vi "R567X_CAN高级功能.vi"(0 "Function":T1(ring), 11 "error in":errorcluster) -> (2 "当前扭矩":dbl, 3 "当前角度":dbl, 4 "完成":bool, 6 "Out_Time":bool, 8 "角度已标定":bool, 10 "扭矩已标定":bool, 15 "error out":errorcluster)   [LabVIEW 2020]
uses:
  Global_Variable/Global.vi
  Libraries/ZLG_CAN/ZLG_CAN.lvlib
  Libraries/S7/S7.lvlib
panel:
  out "Logs":string
  in  "CAN 通道":u32(ring) items=["0", "1"]
  in  "设备类型":u32(ring)=27 items=["PCI5121"=1, "PCI9810"=2, "USBCAN1"=3, "USBCAN2"=4, "PCI9820"=5, "PCI5110"=7, "PC104CAN"=11, "CANETUDP"=12, "PCI9840B"=14, "PC104C2"=15, "PCI9820I"=16, "CANETTCP"=17, "PCIE9221"=24, "PCI5010U"=19, "USBCAN_E_U"=20, "USBCAN_2E_U"=21, "PCI5020U"=22, "PCIE9120I"=27, "PCIE9110I"=28, "PCIE9140I"=29]
  in  "索引":u32(ring) items=["0", "1", "2", "3", "4", "5", "6", "7", "8"]
  in  "波特率":u32(ring)=11 items=["5Kbps", "10Kbps", "20Kbps", "40Kbps", "50Kbps", "80Kbps", "100Kbps", "125Kbps", "200Kbps", "250Kbps", "400Kbps", "500Kbps", "666Kbps", "800Kbps", "1000Kbps"]
  out "B'":i16 format="%x"
  out "B":i16 format="%x"
  out "A":i16 format="%x"
  out "A'":i16 format="%x"
  out "标定成功":bool caption="启动标定成功"
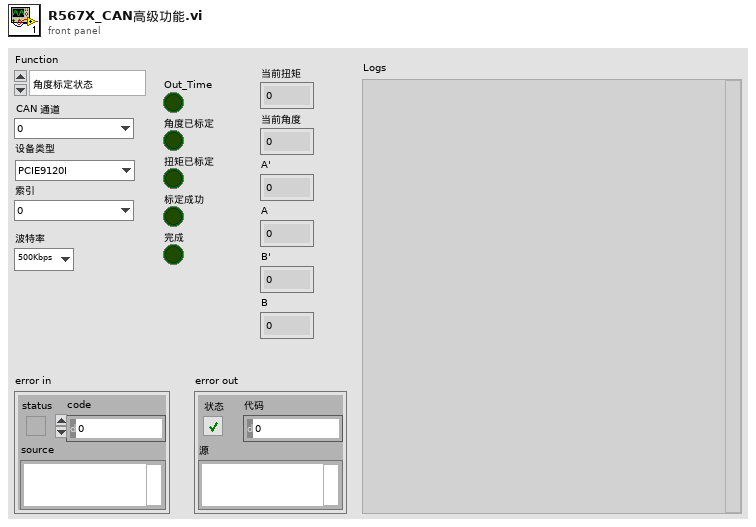
[diagram p1: front panel]
types:
  T1 = enum16{"角度标定状态", "角度标定", "角度标定清除", "扭矩标定状态", "扭矩标定", "扭矩标定清除", "内部软件版本号", "客户软件版本号"}
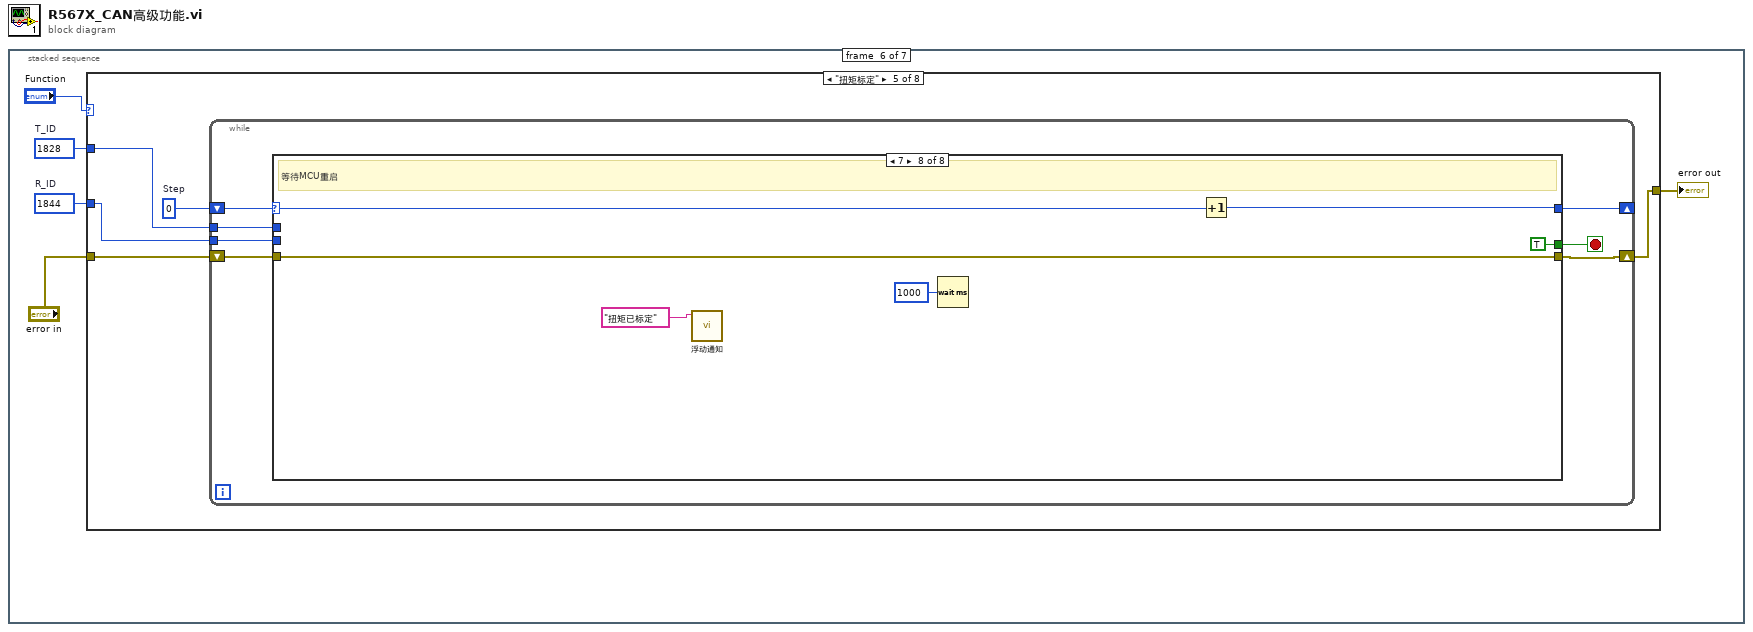
[diagram p0: block diagram]
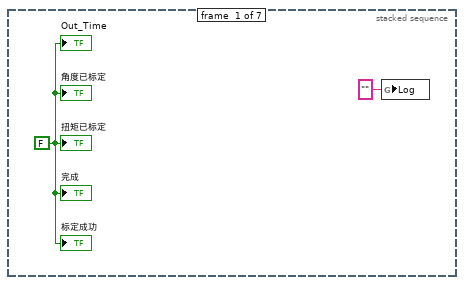
[diagram p2: hidden frame]
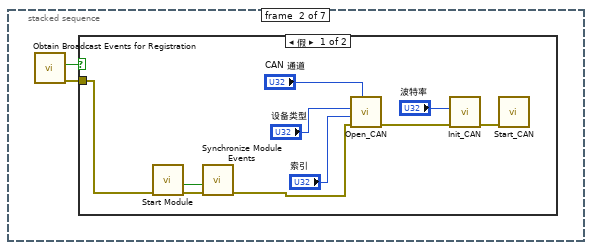
[diagram p3: hidden frame]
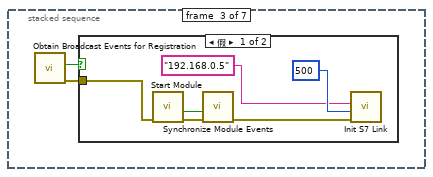
[diagram p5: hidden frame]
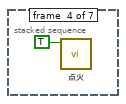
[diagram p7: hidden frame]
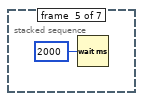
[diagram p8: hidden frame]
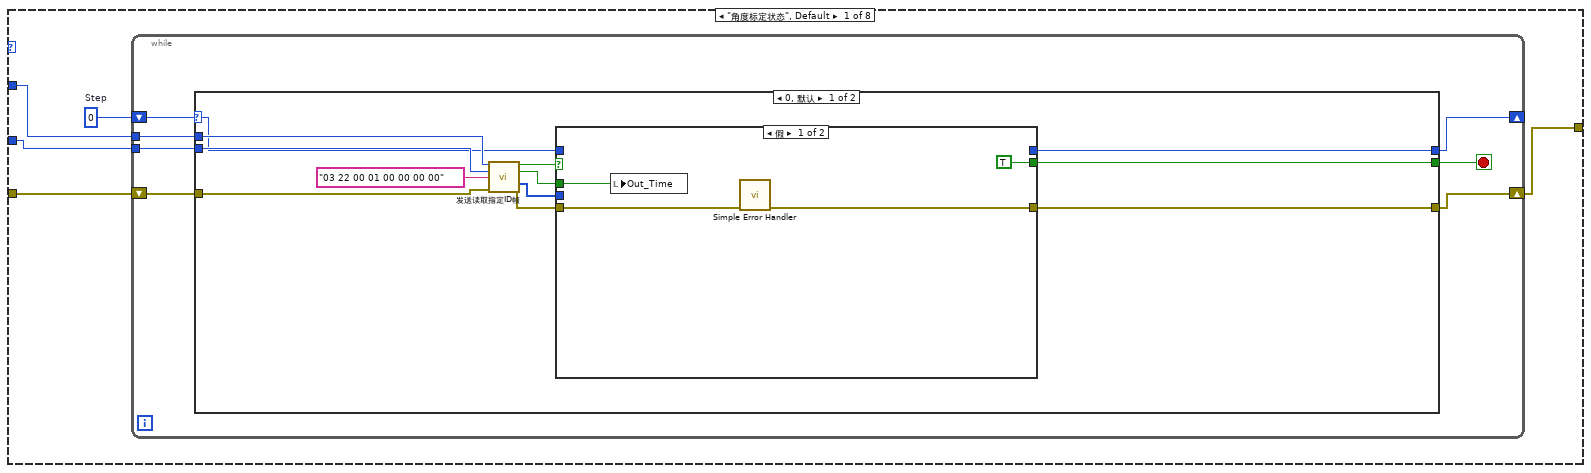
[diagram p9: hidden frame]
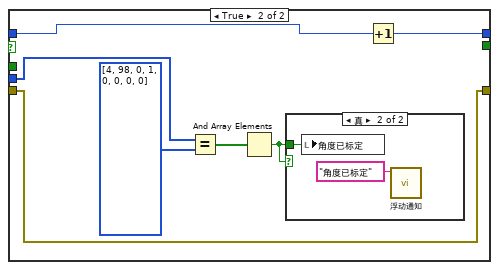
[diagram p10: hidden frame]
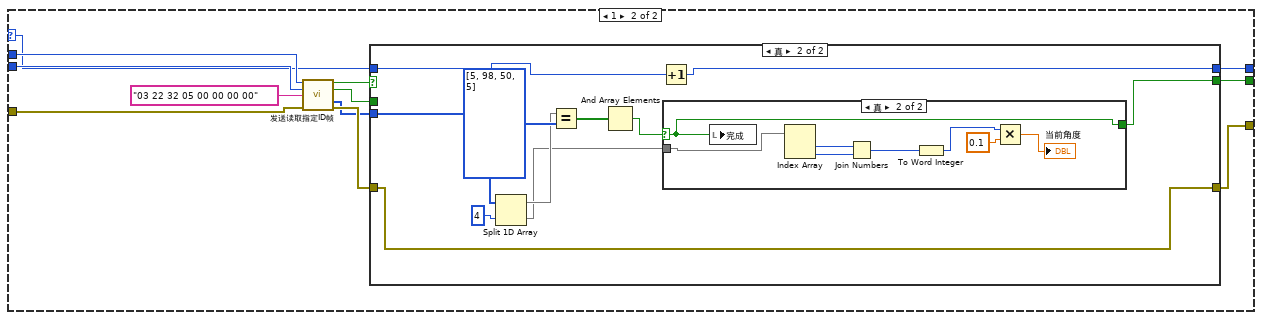
[diagram p12: hidden frame]
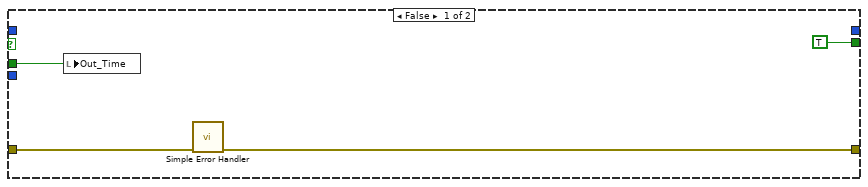
[diagram p13: hidden frame]
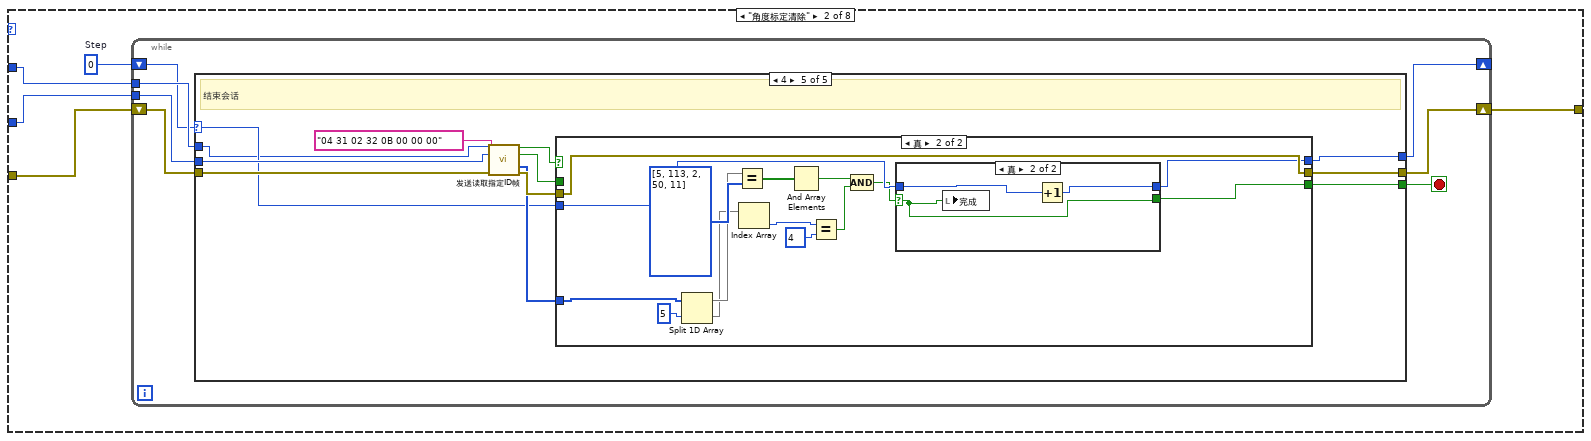
[diagram p15: hidden frame]
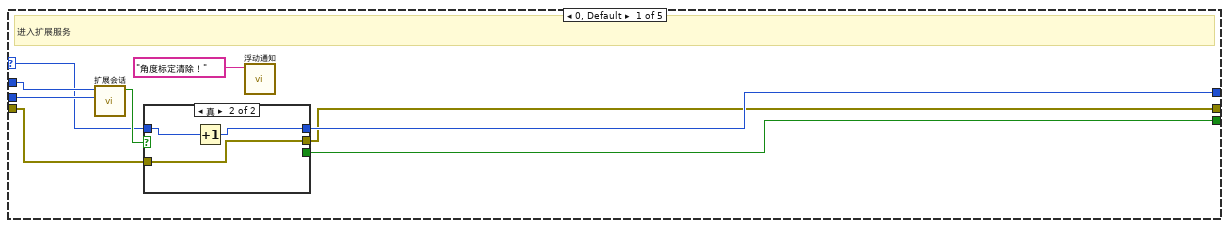
[diagram p16: hidden frame]
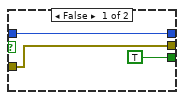
[diagram p17: hidden frame]
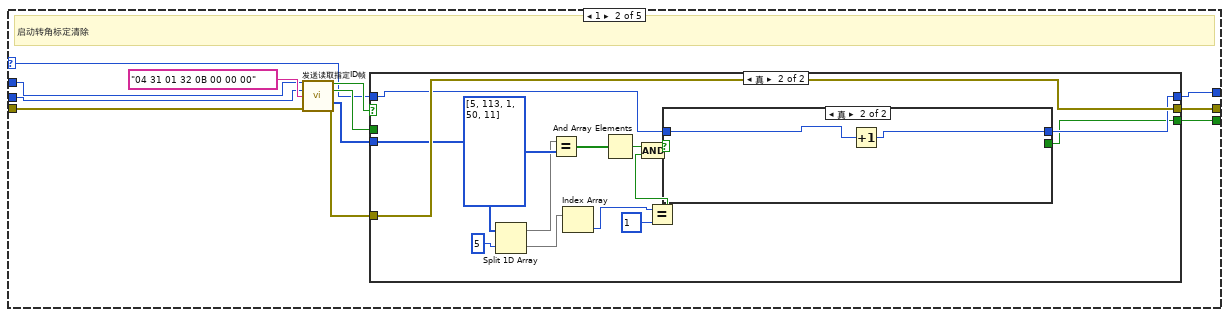
[diagram p18: hidden frame]
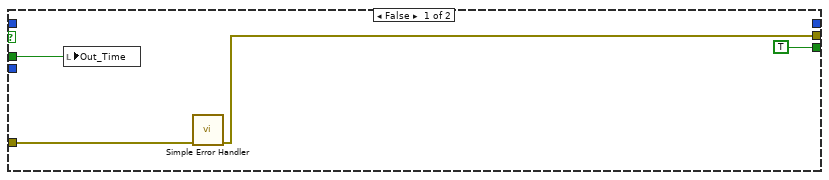
[diagram p19: hidden frame]
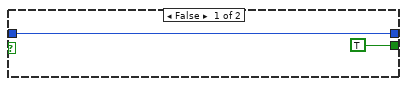
[diagram p20: hidden frame]
diagram:
  n1 = stacked-sequence {
    frame #0 {
      w2 = FALSE ("Out_Time")
      n2 = global write "Global.vi" "Log"("" ("Log")) -> ()
      "Out_Time" <- w2
      "标定成功" <- w2
      "完成" <- w2
      "扭矩已标定" <- w2
      "角度已标定" <- w2
    }
    frame #1 {
      n3 = call "Obtain Broadcast Events for Registration.vi"() -> ("error out"=w3:errorcluster, "Already running?"=w4:bool)  [unwired: 9 in, 1 out]
      n4 = case shown="假" w4 {
        tunnel: w3 -> [w9 _]
        frame False {
          n5 = call "Start Module.vi"("error in (no error)"=w9) -> ("error out"=w10:errorcluster, "Wait for Event Sync?"=w11:bool)  [unwired: 7 in, 2 out]
          n6 = call "Synchronize Module Events.vi"("error in (no error)"=w10, "Wait for Event Sync?"=w11) -> ("error out"=w12:errorcluster)  [unwired: 9 in]
          n7 = call "Open_CAN.vi"("CAN 通道"="CAN 通道", "error in (no error)"=w12, "索引"="索引", "设备类型"="设备类型") -> ("error out"=w13:errorcluster)  [unwired: 7 in]
          n8 = call "Init_CAN.vi"("error in (no error)"=w13, "波特率"="波特率") -> ("error out"=w14:errorcluster)  [unwired: 9 in]
          n9 = call "Start_CAN.vi"("error in (no error)"=w14) -> ()  [unwired: 8 in, 3 out]
        }
        frame True {
        }
      }
    }
    frame #2 {
      n10 = call "Obtain Broadcast Events for Registration.vi"() -> ("error out"=w15:errorcluster, "Already running?"=w16:bool)  [unwired: 9 in, 1 out]
      n11 = case shown="假" w16 {
        tunnel: w15 -> [w17 _]
        frame False {
          n12 = call "Start Module.vi"("error in (no error)"=w17) -> ("error out"=w21:errorcluster, "Wait for Event Sync?"=w20:bool)  [unwired: 7 in, 2 out]
          n13 = call "Synchronize Module Events.vi"("error in (no error)"=w21, "Wait for Event Sync?"=w20) -> ("error out"=w22:errorcluster)  [unwired: 9 in]
          n14 = call "Init S7 Link.vi"("error in (no error)"=w22, "超时"=500, "IP"="192.168.0.5") -> ()  [unwired: 8 in, 1 out]
        }
        frame True {
        }
      }
    }
    frame #3 {
      n15 = call "点火.vi"("点火"=TRUE) -> ()  [unwired: 10 in, 1 out]
    }
    frame #4 {
      n16 = Wait (ms)(milliseconds to wait=u32 2000 ("等待时间（毫秒）")) -> ()  [unwired: 1 out]
    }
    frame #5 {
      w26 = u32 1828  # T_ID
      w25 = u32 1844  # R_ID
      n17 = case shown="\"扭矩标定\"" "Function" {
        tunnel: "error in" -> [w34 w105 w242 w343 w414 w657 w711 w712]
        tunnel: [w32 w104 w241 w341 w413 w656 w711 w712] -> w27
        tunnel: w26 -> [w31 w103 w240 w340 w412 w655 _ _]
        tunnel: w25 -> [w30 w102 w239 w339 w411 w654 _ _]
        frame "角度标定状态", Default {
          w33 = 0  # Step
          n18 = while {
            tunnel: w31 -> [w41]
            tunnel: w30 -> [w39]
            shift-right: [w35] -> _
            shift-left: w33 -> [w38]
            shift-right: [w36] -> w32
            shift-left: w34 -> [w40]
            stop <- w37 stop-if-true
            n19 = case shown="0, 默认" w38 {
              selector: w38 -> [w43 w68]
              tunnel: w41 -> [w53 w78]
              tunnel: w40 -> [w52 w77]
              tunnel: w39 -> [w51 w76]
              tunnel: [w47 w72] -> w37
              tunnel: [w45 w70] -> w36
              tunnel: [w42 w67] -> w35
              frame 0, Default {
                n20 = call "发送读取指定ID帧.vi"("T_ID"=w53, "R_ID"=w51, "CAN_Frame"="03 22 00 01 00 00 00 00", "error in (no error)"=w52) -> ("OK"=w49:bool, "Out_Time"=w48:bool, "Recive"=w44:u8[], "error out"=w46:errorcluster)  [unwired: 7 in, 1 out]
                n21 = case shown="假" w49 {
                  tunnel: w48 -> [w57 _]
                  tunnel: [TRUE _] -> w47
                  tunnel: w46 -> [w55 w64]
                  tunnel: [w54 w64] -> w45
                  tunnel: w44 -> [_ w63]
                  tunnel: w43 -> [_ w60]
                  tunnel: [_ w59] -> w42
                  frame False {
                    n22 = local write "Out_Time"(w57) -> ()
                    n23 = call <vilib>:"Simple Error Handler.vi"("error in (no error)"=w55) -> ("error out"=w54:errorcluster)  [unwired: 4 in, 4 out]
                  }
                  frame True {
                    n24 = Equal?(x=w63, y=u8[] [4, 98, 0, 1, 0, 0, 0, 0]) -> (x = y?=w61:bool[])
                    n25 = And Array Elements(Boolean array=w61) -> (logical AND=w58:bool)
                    n26 = case shown="真" w58 {
                      tunnel: w58 -> [_ w66]
                      frame False {
                      }
                      frame True {
                        n27 = local write "角度已标定"(w66) -> ()
                        n28 = call "浮动通知.vi"("通知内容"="角度已标定") -> ()  [unwired: 11 in]
                      }
                    }
                    n29 = Increment(x=w60) -> (x+1=w59:i32)
                  }
                }
              }
              frame 1 {
                n30 = call "发送读取指定ID帧.vi"("T_ID"=w78, "R_ID"=w76, "CAN_Frame"="03 22 32 05 00 00 00 00", "error in (no error)"=w77) -> ("OK"=w74:bool, "Out_Time"=w73:bool, "Recive"=w69:u8[], "error out"=w71:errorcluster)  [unwired: 7 in, 1 out]
                n31 = case shown="真" w74 {
                  tunnel: w73 -> [w82 _]
                  tunnel: [TRUE w83] -> w72
                  tunnel: w71 -> [w80 w93]
                  tunnel: [w79 w93] -> w70
                  tunnel: w69 -> [_ w88]
                  tunnel: w68 -> [_ w90]
                  tunnel: [_ w89] -> w67
                  frame False {
                    n32 = local write "Out_Time"(w82) -> ()
                    n33 = call <vilib>:"Simple Error Handler.vi"("error in (no error)"=w80) -> ("error out"=w79:errorcluster)  [unwired: 4 in, 4 out]
                  }
                  frame True {
                    n34 = Split 1D Array(array=w88, index=4 ("索引")) -> (first subarray=w86:u8[], second subarray=w85:u8[])
                    n35 = Equal?(x=w86, y=u8[] [5, 98, 50, 5]) -> (x = y?=w91:bool[])
                    n36 = And Array Elements(Boolean array=w91) -> (logical AND=w84:bool)
                    n37 = Increment(x=w90) -> (x+1=w89:i32)
                    n38 = case shown="真" w84 {
                      selector: w84 -> [_ w94]
                      tunnel: w85 -> [_ w101]
                      tunnel: [_ w94] -> w83
                      frame False {
                      }
                      frame True {
                        n39 = local write "完成"(w94) -> ()
                        n40 = Index Array(array=w101) -> (element #1=w99:u8, element #2=w100:u8)  [unwired: 2 in]
                        n41 = Join Numbers(hi=w99, lo=w100) -> ((hi.lo)=w96:u16)
                        n42 = To Word Integer(number=w96) -> (16bit integer=w95:i16)
                        n43 = Multiply(x=w95, y=0.1) -> (x*y=→"当前角度":dbl)
                      }
                    }
                  }
                }
              }
            }
          }
        }
        frame "角度标定清除" {
          w106 = 0  # Step
          n44 = while {
            tunnel: w103 -> [w113]
            tunnel: w102 -> [w111]
            shift-right: [w107] -> _
            shift-left: w106 -> [w110]
            shift-right: [w108] -> w104
            shift-left: w105 -> [w112]
            stop <- w109 stop-if-true
            n45 = case shown="4" w110 {
              selector: w110 -> [w119 w133 w166 w172 w208]
              tunnel: w113 -> [w122 w132 _ w171 w207]
              tunnel: w112 -> [w116 w134 w164 w173 w209]
              tunnel: w111 -> [w121 w135 _ w174 w210]
              tunnel: [w117 w130 _ w169 w205] -> w109
              tunnel: [w115 w129 w164 w168 w204] -> w108
              tunnel: [w118 w131 w165 w170 w206] -> w107
              frame 0, Default {
                # "进入扩展服务"
                n46 = call "扩展会话.vi"("R_ID"=w121, "T_ID"=w122) -> ("OK"=w120:bool)  [unwired: 8 in, 1 out]
                n47 = case shown="真" w120 {
                  tunnel: w119 -> [w125 w128]
                  tunnel: [w125 w127] -> w118
                  tunnel: [TRUE _] -> w117
                  tunnel: [w123 w126] -> w115
                  tunnel: w116 -> [w123 w126]
                  frame False {
                  }
                  frame True {
                    n48 = Increment(x=w128) -> (x+1=w127:i32)
                  }
                }
                n49 = call "浮动通知.vi"("通知内容"="角度标定清除！") -> ()  [unwired: 11 in]
              }
              frame 1 {
                # "启动转角标定清除"
                n50 = call "发送读取指定ID帧.vi"("T_ID"=w132, "R_ID"=w135, "CAN_Frame"="04 31 01 32 0B 00 00 00", "error in (no error)"=w134) -> ("OK"=w140:bool, "Out_Time"=w139:bool, "Recive"=w137:u8[], "error out"=w138:errorcluster)  [unwired: 7 in, 1 out]
                n51 = case shown="真" w140 {
                  tunnel: w139 -> [w144 _]
                  tunnel: [TRUE w150] -> w130
                  tunnel: w138 -> [w142 w159]
                  tunnel: [w141 w159] -> w129
                  tunnel: w137 -> [_ w156]
                  tunnel: w133 -> [_ w152]
                  tunnel: [_ w151] -> w131
                  frame False {
                    n52 = local write "Out_Time"(w144) -> ()
                    n53 = call <vilib>:"Simple Error Handler.vi"("error in (no error)"=w142) -> ("error out"=w141:errorcluster)  [unwired: 4 in, 4 out]
                  }
                  frame True {
                    n54 = Split 1D Array(array=w156, index=5 ("索引")) -> (first subarray=w154:u8[], second subarray=w147:u8[])
                    n55 = Equal?(x=w154, y=u8[] [5, 113, 1, 50, 11]) -> (x = y?=w157:bool[])
                    n56 = Index Array(array=w147) -> (element=w149:u8)  [unwired: 1 in]
                    n57 = And Array Elements(Boolean array=w157) -> (logical AND=w153:bool)
                    n58 = Equal?(x=w149, y=u8 1) -> (x = y?=w145:bool)
                    n59 = Compound Arithmetic op=AND ("复合运算")(w153, w145) -> (w146:bool)
                    n60 = case shown="真" w146 {
                      tunnel: w152 -> [w161 w163]
                      tunnel: [w161 w162] -> w151
                      tunnel: [TRUE _] -> w150
                      frame False {
                      }
                      frame True {
                        n61 = Increment(x=w163) -> (x+1=w162:i32)
                      }
                    }
                  }
                }
              }
              frame 2 {
                # "等待角度标定清除"
                n62 = Wait (ms)(milliseconds to wait=u32 200 ("等待时间（毫秒）")) -> ()  [unwired: 1 out]
                n63 = Increment(x=w166) -> (x+1=w165:i32)
              }
              frame 3 {
                # "获取角度标定清除结果"
                n64 = call "发送读取指定ID帧.vi"("T_ID"=w171, "R_ID"=w174, "CAN_Frame"="04 31 03 32 0B 00 00 00", "error in (no error)"=w173) -> ("OK"=w179:bool, "Out_Time"=w178:bool, "Recive"=w176:u8[], "error out"=w177:errorcluster)  [unwired: 7 in, 1 out]
                n65 = case shown="真" w179 {
                  tunnel: w178 -> [w183 _]
                  tunnel: [TRUE w189] -> w169
                  tunnel: w177 -> [w181 w198]
                  tunnel: [w180 w198] -> w168
                  tunnel: w176 -> [_ w195]
                  tunnel: w172 -> [_ w191]
                  tunnel: [_ w190] -> w170
                  frame False {
                    n66 = local write "Out_Time"(w183) -> ()
                    n67 = call <vilib>:"Simple Error Handler.vi"("error in (no error)"=w181) -> ("error out"=w180:errorcluster)  [unwired: 4 in, 4 out]
                  }
                  frame True {
                    n68 = Split 1D Array(array=w195, index=5 ("索引")) -> (first subarray=w193:u8[], second subarray=w186:u8[])
                    n69 = Equal?(x=w193, y=u8[] [5, 113, 3, 50, 11]) -> (x = y?=w196:bool[])
                    n70 = Index Array(array=w186) -> (element=w188:u8)  [unwired: 1 in]
                    n71 = And Array Elements(Boolean array=w196) -> (logical AND=w192:bool)
                    n72 = Equal?(x=w188, y=u8 2) -> (x = y?=w184:bool)
                    n73 = Compound Arithmetic op=AND ("复合运算")(w184, w192) -> (w185:bool)
                    n74 = case shown="真" w185 {
                      selector: w185 -> [_ w201]
                      tunnel: w191 -> [w200 w203]
                      tunnel: [w200 w202] -> w190
                      tunnel: [TRUE _] -> w189
                      frame False {
                      }
                      frame True {
                        n75 = Increment(x=w203) -> (x+1=w202:i32)
                        n76 = local write "标定成功"(w201) -> ()
                      }
                    }
                  }
                }
              }
              frame 4 {
                # "结束会话"
                n77 = call "发送读取指定ID帧.vi"("T_ID"=w207, "R_ID"=w210, "CAN_Frame"="04 31 02 32 0B 00 00 00", "error in (no error)"=w209) -> ("OK"=w215:bool, "Out_Time"=w214:bool, "Recive"=w212:u8[], "error out"=w213:errorcluster)  [unwired: 7 in, 1 out]
                n78 = case shown="真" w215 {
                  tunnel: w214 -> [w219 _]
                  tunnel: [TRUE w227] -> w205
                  tunnel: w213 -> [w217 w234]
                  tunnel: [w216 w234] -> w204
                  tunnel: w212 -> [_ w231]
                  tunnel: w208 -> [_ w223]
                  tunnel: [_ w222] -> w206
                  frame False {
                    n79 = local write "Out_Time"(w219) -> ()
                    n80 = call <vilib>:"Simple Error Handler.vi"("error in (no error)"=w217) -> ("error out"=w216:errorcluster)  [unwired: 4 in, 4 out]
                  }
                  frame True {
                    n81 = Split 1D Array(array=w231, index=5 ("索引")) -> (first subarray=w229:u8[], second subarray=w224:u8[])
                    n82 = Equal?(x=w229, y=u8[] [5, 113, 2, 50, 11]) -> (x = y?=w232:bool[])
                    n83 = Index Array(array=w224) -> (element=w226:u8)  [unwired: 1 in]
                    n84 = And Array Elements(Boolean array=w232) -> (logical AND=w228:bool)
                    n85 = Equal?(x=w226, y=u8 4) -> (x = y?=w220:bool)
                    n86 = Compound Arithmetic op=AND ("复合运算")(w228, w220) -> (w221:bool)
                    n87 = case shown="真" w221 {
                      selector: w221 -> [_ w236]
                      tunnel: [TRUE w236] -> w227
                      tunnel: w223 -> [_ w238]
                      tunnel: [_ w237] -> w222
                      frame False {
                      }
                      frame True {
                        n88 = local write "完成"(w236) -> ()
                        n89 = Increment(x=w238) -> (x+1=w237:i32)
                      }
                    }
                  }
                }
              }
            }
          }
        }
        frame "角度标定" {
          w243 = 0  # Step
          n90 = while {
            tunnel: w240 -> [w250]
            tunnel: w239 -> [w248]
            shift-right: [w244] -> _
            shift-left: w243 -> [w247]
            shift-right: [w245] -> w241
            shift-left: w242 -> [w249]
            stop <- w246 stop-if-true
            n91 = case shown="0, 2, 默认" w247 {
              selector: w247 -> [w256 w270 w305]
              tunnel: w250 -> [w259 w269 w304]
              tunnel: w249 -> [w253 w271 w306]
              tunnel: w248 -> [w258 w272 w307]
              tunnel: [w254 w267 w302] -> w246
              tunnel: [w252 w266 w301] -> w245
              tunnel: [w255 w268 w303] -> w244
              frame 0, 2, Default {
                # "进入扩展服务"
                n92 = call "扩展会话.vi"("R_ID"=w258, "T_ID"=w259) -> ("OK"=w257:bool)  [unwired: 8 in, 1 out]
                n93 = case shown="真" w257 {
                  tunnel: w256 -> [w262 w265]
                  tunnel: [w262 w264] -> w255
                  tunnel: [TRUE _] -> w254
                  tunnel: [w260 w263] -> w252
                  tunnel: w253 -> [w260 w263]
                  frame False {
                  }
                  frame True {
                    n94 = Increment(x=w265) -> (x+1=w264:i32)
                  }
                }
                n95 = call "浮动通知.vi"("通知内容"="角度标定……") -> ()  [unwired: 11 in]
              }
              frame 1 {
                # "启动转角标定"
                n96 = call "发送读取指定ID帧.vi"("T_ID"=w269, "R_ID"=w272, "CAN_Frame"="04 31 01 AC CF 00 00 00", "error in (no error)"=w271) -> ("OK"=w277:bool, "Out_Time"=w276:bool, "Recive"=w274:u8[], "error out"=w275:errorcluster)  [unwired: 7 in, 1 out]
                n97 = case shown="真" w277 {
                  tunnel: w276 -> [w281 _]
                  tunnel: [TRUE w287] -> w267
                  tunnel: w275 -> [w279 w296]
                  tunnel: [w278 w296] -> w266
                  tunnel: w274 -> [_ w293]
                  tunnel: w270 -> [_ w289]
                  tunnel: [_ w288] -> w268
                  frame False {
                    n98 = local write "Out_Time"(w281) -> ()
                    n99 = call <vilib>:"Simple Error Handler.vi"("error in (no error)"=w279) -> ("error out"=w278:errorcluster)  [unwired: 4 in, 4 out]
                  }
                  frame True {
                    n100 = Split 1D Array(array=w293, index=5 ("索引")) -> (first subarray=w291:u8[], second subarray=w284:u8[])
                    n101 = Equal?(x=w291, y=u8[] [5, 113, 1, 172, 207]) -> (x = y?=w294:bool[])
                    n102 = Index Array(array=w284) -> (element=w286:u8)  [unwired: 1 in]
                    n103 = And Array Elements(Boolean array=w294) -> (logical AND=w290:bool)
                    n104 = Equal?(x=w286, y=u8 1) -> (x = y?=w282:bool)
                    n105 = Compound Arithmetic op=AND ("复合运算")(w290, w282) -> (w283:bool)
                    n106 = case shown="真" w283 {
                      tunnel: w289 -> [w298 w300]
                      tunnel: [w298 w299] -> w288
                      tunnel: [TRUE _] -> w287
                      frame False {
                      }
                      frame True {
                        n107 = Increment(x=w300) -> (x+1=w299:i32)
                      }
                    }
                  }
                }
              }
              frame 3 {
                # "获取角度标定结果"
                n108 = call "发送读取指定ID帧.vi"("T_ID"=w304, "R_ID"=w307, "CAN_Frame"="04 31 03 AC CF 00 00 00", "error in (no error)"=w306) -> ("OK"=w312:bool, "Out_Time"=w311:bool, "Recive"=w309:u8[], "error out"=w310:errorcluster)  [unwired: 7 in, 1 out]
                n109 = case shown="真" w312 {
                  tunnel: w311 -> [w316 _]
                  tunnel: [TRUE w322] -> w302
                  tunnel: w310 -> [w314 w331]
                  tunnel: [w313 w331] -> w301
                  tunnel: w309 -> [_ w328]
                  tunnel: w305 -> [_ w324]
                  tunnel: [_ w323] -> w303
                  frame False {
                    n110 = local write "Out_Time"(w316) -> ()
                    n111 = call <vilib>:"Simple Error Handler.vi"("error in (no error)"=w314) -> ("error out"=w313:errorcluster)  [unwired: 4 in, 4 out]
                  }
                  frame True {
                    n112 = Split 1D Array(array=w328, index=5 ("索引")) -> (first subarray=w326:u8[], second subarray=w319:u8[])
                    n113 = Index Array(array=w319) -> (element=w321:u8)  [unwired: 1 in]
                    n114 = Equal?(x=w326, y=u8[] [5, 113, 3, 172, 207]) -> (x = y?=w329:bool[])
                    n115 = And Array Elements(Boolean array=w329) -> (logical AND=w325:bool)
                    n116 = Equal?(x=w321, y=u8 1) -> (x = y?=w317:bool)
                    n117 = Compound Arithmetic op=AND ("复合运算")(w325, w317) -> (w318:bool)
                    n118 = case shown="真" w318 {
                      selector: w318 -> [_ w335]
                      tunnel: w324 -> [w333 w338]
                      tunnel: [w333 w337] -> w323
                      tunnel: [TRUE TRUE] -> w322
                      frame False {
                      }
                      frame True {
                        n119 = local write "完成"(w335) -> ()
                        n120 = Increment(x=w338) -> (x+1=w337:i32)
                        n121 = call "浮动通知.vi"("通知内容"="角度标定成功") -> ()  [unwired: 11 in]
                      }
                    }
                  }
                }
              }
            }
          }
        }
        frame "扭矩标定状态" {
          w342 = 0  # Step
          n122 = while {
            shift-right: [w346] -> _
            shift-left: w342 -> [w349]
            shift-right: [w347] -> w341
            shift-left: w343 -> [w350]
            tunnel: w340 -> [w345]
            tunnel: w339 -> [w344]
            stop <- w348 stop-if-true
            n123 = case shown="1" w349 {
              selector: w349 -> [w352 w377]
              tunnel: w345 -> [w362 w387]
              tunnel: w350 -> [w361 w386]
              tunnel: w344 -> [w360 w385]
              tunnel: [w356 w381] -> w348
              tunnel: [w354 w379] -> w347
              tunnel: [w351 w376] -> w346
              frame 0, Default {
                n124 = call "发送读取指定ID帧.vi"("T_ID"=w362, "R_ID"=w360, "CAN_Frame"="03 22 00 05 00 00 00 00", "error in (no error)"=w361) -> ("OK"=w358:bool, "Out_Time"=w357:bool, "Recive"=w353:u8[], "error out"=w355:errorcluster)  [unwired: 7 in, 1 out]
                n125 = case shown="真" w358 {
                  tunnel: w357 -> [w366 _]
                  tunnel: [TRUE _] -> w356
                  tunnel: w355 -> [w364 w373]
                  tunnel: [w363 w373] -> w354
                  tunnel: w353 -> [_ w372]
                  tunnel: w352 -> [_ w369]
                  tunnel: [_ w368] -> w351
                  frame False {
                    n126 = local write "Out_Time"(w366) -> ()
                    n127 = call <vilib>:"Simple Error Handler.vi"("error in (no error)"=w364) -> ("error out"=w363:errorcluster)  [unwired: 4 in, 4 out]
                  }
                  frame True {
                    n128 = Equal?(x=w372, y=u8[] [4, 98, 0, 5, 0, 0, 0, 0]) -> (x = y?=w370:bool[])
                    n129 = And Array Elements(Boolean array=w370) -> (logical AND=w367:bool)
                    n130 = case shown="真" w367 {
                      tunnel: w367 -> [_ w375]
                      frame False {
                      }
                      frame True {
                        n131 = local write "扭矩已标定"(w375) -> ()
                        n132 = call "浮动通知.vi"("通知内容"="扭矩已标定") -> ()  [unwired: 11 in]
                      }
                    }
                    n133 = Increment(x=w369) -> (x+1=w368:i32)
                  }
                }
              }
              frame 1 {
                n134 = call "发送读取指定ID帧.vi"("T_ID"=w387, "R_ID"=w385, "CAN_Frame"="03 22 32 02 00 00 00 00", "error in (no error)"=w386) -> ("OK"=w383:bool, "Out_Time"=w382:bool, "Recive"=w378:u8[], "error out"=w380:errorcluster)  [unwired: 7 in, 1 out]
                n135 = case shown="真" w383 {
                  tunnel: w382 -> [w391 _]
                  tunnel: [TRUE w392] -> w381
                  tunnel: w380 -> [w389 w402]
                  tunnel: [w388 w402] -> w379
                  tunnel: w378 -> [_ w397]
                  tunnel: w377 -> [_ w399]
                  tunnel: [_ w398] -> w376
                  frame False {
                    n136 = local write "Out_Time"(w391) -> ()
                    n137 = call <vilib>:"Simple Error Handler.vi"("error in (no error)"=w389) -> ("error out"=w388:errorcluster)  [unwired: 4 in, 4 out]
                  }
                  frame True {
                    n138 = Split 1D Array(array=w397, index=4 ("索引")) -> (first subarray=w395:u8[], second subarray=w394:u8[])
                    n139 = Equal?(x=w395, y=u8[] [5, 98, 50, 2]) -> (x = y?=w400:bool[])
                    n140 = And Array Elements(Boolean array=w400) -> (logical AND=w393:bool)
                    n141 = Increment(x=w399) -> (x+1=w398:i32)
                    n142 = case shown="真" w393 {
                      selector: w393 -> [_ w403]
                      tunnel: w394 -> [_ w410]
                      tunnel: [_ w403] -> w392
                      frame False {
                      }
                      frame True {
                        n143 = local write "完成"(w403) -> ()
                        n144 = Index Array(array=w410) -> (element #1=w408:u8, element #2=w409:u8)  [unwired: 2 in]
                        n145 = Join Numbers(hi=w408, lo=w409) -> ((hi.lo)=w405:u16)
                        n146 = To Word Integer(number=w405) -> (16bit integer=w404:i16)
                        n147 = Multiply(x=w404, y=0.0009765625) -> (x*y=→"当前扭矩":dbl)
                      }
                    }
                  }
                }
              }
            }
          }
        }
        frame "扭矩标定" {
          w415 = 0  # Step
          n148 = while {
            tunnel: w412 -> [w422]
            tunnel: w411 -> [w420]
            shift-right: [w416] -> _
            shift-left: w415 -> [w419]
            shift-right: [w417] -> w413
            shift-left: w414 -> [w421]
            stop <- w418 stop-if-true
            n149 = case shown="7" w419 {
              selector: w419 -> [w425 w463 w501 w517 w550 w582 w619 w651]
              tunnel: w422 -> [w435 w473 w508 w533 w566 w592 w629 _]
              tunnel: w421 -> [w434 w472 w506 w523 w556 w591 w628 w653]
              tunnel: w420 -> [w433 w471 w507 w532 w565 w590 w627 _]
              tunnel: [w429 w467 w502 w515 w548 w586 w623 TRUE] -> w418
              tunnel: [w427 w465 w503 w519 w552 w584 w621 w653] -> w417
              tunnel: [w424 w462 w500 w516 w549 w581 w618 w650] -> w416
              frame 0, Default {
                # "读取T1原始值A"
                n150 = call "浮动通知.vi"("通知内容"="扭矩标定……") -> ()  [unwired: 11 in]
                n151 = call "发送读取指定ID帧.vi"("T_ID"=w435, "R_ID"=w433, "CAN_Frame"="03 22 07 00 00 00 00 00", "error in (no error)"=w434) -> ("OK"=w431:bool, "Out_Time"=w430:bool, "Recive"=w426:u8[], "error out"=w428:errorcluster)  [unwired: 7 in, 1 out]
                n152 = case shown="真" w431 {
                  tunnel: w430 -> [w439 _]
                  tunnel: [TRUE w440] -> w429
                  tunnel: w428 -> [w437 w450]
                  tunnel: [w436 w450] -> w427
                  tunnel: w426 -> [_ w447]
                  tunnel: w425 -> [_ w442]
                  tunnel: [_ w441] -> w424
                  frame False {
                    n153 = local write "Out_Time"(w439) -> ()
                    n154 = call <vilib>:"Simple Error Handler.vi"("error in (no error)"=w437) -> ("error out"=w436:errorcluster)  [unwired: 4 in, 4 out]
                  }
                  frame True {
                    n155 = Split 1D Array(array=w447, index=4 ("索引")) -> (first subarray=w445:u8[], second subarray=w444:u8[])
                    n156 = Equal?(x=w445, y=u8[] [5, 98, 7, 0]) -> (x = y?=w448:bool[])
                    n157 = And Array Elements(Boolean array=w448) -> (logical AND=w443:bool)
                    n158 = case shown="真" w443 {
                      tunnel: w444 -> [_ w461]
                      tunnel: w442 -> [w451 w454]
                      tunnel: [w451 w453] -> w441
                      tunnel: [TRUE _] -> w440
                      frame False {
                      }
                      frame True {
                        n159 = Index Array(array=w461) -> (element #1=w459:u8, element #2=w460:u8)  [unwired: 2 in]
                        n160 = Join Numbers(hi=w459, lo=w460) -> ((hi.lo)=w458:u16)
                        n161 = Increment(x=w454) -> (x+1=w453:i32)
                        n162 = To Word Integer(number=w458) -> (16bit integer=w457:i16)
                        "A" <- w457
                        n163 = Subtract(x=i16 16384 ("16位整型"), y=w457) -> (x-y=→"A'":i16)
                      }
                    }
                  }
                }
              }
              frame 1 {
                # "读取T2原始值B"
                n164 = call "发送读取指定ID帧.vi"("T_ID"=w473, "R_ID"=w471, "CAN_Frame"="03 22 07 01 00 00 00 00", "error in (no error)"=w472) -> ("OK"=w469:bool, "Out_Time"=w468:bool, "Recive"=w464:u8[], "error out"=w466:errorcluster)  [unwired: 7 in, 1 out]
                n165 = case shown="真" w469 {
                  tunnel: w468 -> [w477 _]
                  tunnel: [TRUE w478] -> w467
                  tunnel: w466 -> [w475 w488]
                  tunnel: [w474 w488] -> w465
                  tunnel: w464 -> [_ w485]
                  tunnel: w463 -> [_ w480]
                  tunnel: [_ w479] -> w462
                  frame False {
                    n166 = local write "Out_Time"(w477) -> ()
                    n167 = call <vilib>:"Simple Error Handler.vi"("error in (no error)"=w475) -> ("error out"=w474:errorcluster)  [unwired: 4 in, 4 out]
                  }
                  frame True {
                    n168 = Split 1D Array(array=w485, index=4 ("索引")) -> (first subarray=w483:u8[], second subarray=w482:u8[])
                    n169 = Equal?(x=w483, y=u8[] [5, 98, 7, 1]) -> (x = y?=w486:bool[])
                    n170 = And Array Elements(Boolean array=w486) -> (logical AND=w481:bool)
                    n171 = case shown="真" w481 {
                      tunnel: w482 -> [_ w499]
                      tunnel: w480 -> [w489 w492]
                      tunnel: [w489 w491] -> w479
                      tunnel: [TRUE _] -> w478
                      frame False {
                      }
                      frame True {
                        n172 = Increment(x=w492) -> (x+1=w491:i32)
                        n173 = Index Array(array=w499) -> (element #1=w497:u8, element #2=w498:u8)  [unwired: 2 in]
                        n174 = Join Numbers(hi=w497, lo=w498) -> ((hi.lo)=w496:u16)
                        n175 = To Word Integer(number=w496) -> (16bit integer=w495:i16)
                        "B" <- w495
                        n176 = Subtract(x=i16 16384 ("16位整型"), y=w495) -> (x-y=→"B'":i16)
                      }
                    }
                  }
                }
              }
              frame 2 {
                # "进入扩展会话"
                n177 = call "扩展会话.vi"("error in"=w506, "R_ID"=w507, "T_ID"=w508) -> ("error out"=w504:errorcluster, "OK"=w505:bool)  [unwired: 7 in]
                n178 = case shown="假" w505 {
                  tunnel: w504 -> [w511 w514]
                  tunnel: [w511 w514] -> w503
                  tunnel: [TRUE _] -> w502
                  tunnel: w501 -> [w509 w513]
                  tunnel: [w509 w512] -> w500
                  frame False {
                  }
                  frame True {
                    n179 = Increment(x=w513) -> (x+1=w512:i32)
                  }
                }
              }
              frame 3 {
                w527 = i16 2 ("宽度(-)")
                # "写入T1标定值A'"
                n180 = local read "A'"() -> (w530:i16)
                n181 = Split Number(x=w530) -> (hi(x)=w529:u8, lo(x)=w528:u8)
                n182 = Number To Hexadecimal String(1:w527, 2:w529) -> (0:w526:string)
                n183 = Number To Hexadecimal String(1:w527, 2:w528) -> (0:w525:string)
                n184 = Format Into String(format string="10 09 31 01 33 01 %s %s" ("格式字符串"), w526, w525) -> (resulting string=w524:string)  [unwired: 2 in, 1 out]
                n185 = call "发送读取指定ID帧.vi"("T_ID"=w533, "R_ID"=w532, "CAN_Frame"=w524, "error in (no error)"=w523) -> ("OK"=w522:bool, "Out_Time"=w521:bool, "Recive"=w518:u8[], "error out"=w520:errorcluster)  [unwired: 7 in, 1 out]
                n186 = case shown="真" w522 {
                  tunnel: w521 -> [w536 _]
                  tunnel: w520 -> [w535 w538]
                  tunnel: [w534 w538] -> w519
                  tunnel: w518 -> [_ w542]
                  tunnel: w517 -> [_ w540]
                  tunnel: [_ w539] -> w516
                  tunnel: [_ w537] -> w515
                  frame False {
                    n187 = local write "Out_Time"(w536) -> ()
                    n188 = call <vilib>:"Simple Error Handler.vi"("error in (no error)"=w535) -> ("error out"=w534:errorcluster)  [unwired: 4 in, 4 out]
                  }
                  frame True {
                    n189 = Equal?(x=w542, y=u8[] [48, 8, 20, 0, 0, 0, 0, 0]) -> (x = y?=w544:bool[])
                    n190 = And Array Elements(Boolean array=w544) -> (logical AND=w541:bool)
                    n191 = case shown="真" w541 {
                      tunnel: w540 -> [_ w547]
                      tunnel: [_ w546] -> w539
                      tunnel: [TRUE _] -> w537
                      frame False {
                      }
                      frame True {
                        n192 = Increment(x=w547) -> (x+1=w546:i32)
                      }
                    }
                  }
                }
              }
              frame 4 {
                w560 = i16 2 ("宽度(-)")
                # "写入T2标定值B'"
                n193 = local read "B'"() -> (w563:i16)
                n194 = Split Number(x=w563) -> (hi(x)=w562:u8, lo(x)=w561:u8)
                n195 = Number To Hexadecimal String(1:w560, 2:w562) -> (0:w559:string)
                n196 = Number To Hexadecimal String(1:w560, 2:w561) -> (0:w558:string)
                n197 = Format Into String(format string="21 %s %s 00 00 00 00 00" ("格式字符串"), w559, w558) -> (resulting string=w557:string)  [unwired: 2 in, 1 out]
                n198 = call "发送读取指定ID帧.vi"("T_ID"=w566, "R_ID"=w565, "CAN_Frame"=w557, "error in (no error)"=w556) -> ("OK"=w555:bool, "Out_Time"=w554:bool, "Recive"=w551:u8[], "error out"=w553:errorcluster)  [unwired: 7 in, 1 out]
                n199 = case shown="真" w555 {
                  tunnel: w554 -> [w569 _]
                  tunnel: w553 -> [w568 w571]
                  tunnel: [w567 w571] -> w552
                  tunnel: w551 -> [_ w575]
                  tunnel: w550 -> [_ w573]
                  tunnel: [_ w572] -> w549
                  tunnel: [_ w570] -> w548
                  frame False {
                    n200 = local write "Out_Time"(w569) -> ()
                    n201 = call <vilib>:"Simple Error Handler.vi"("error in (no error)"=w568) -> ("error out"=w567:errorcluster)  [unwired: 4 in, 4 out]
                  }
                  frame True {
                    n202 = Equal?(x=w575, y=u8[] [5, 113, 1, 51, 1, 1, 0, 0]) -> (x = y?=w577:bool[])
                    n203 = And Array Elements(Boolean array=w577) -> (logical AND=w574:bool)
                    n204 = case shown="真" w574 {
                      tunnel: w573 -> [_ w580]
                      tunnel: [_ w579] -> w572
                      tunnel: [TRUE _] -> w570
                      frame False {
                      }
                      frame True {
                        n205 = Increment(x=w580) -> (x+1=w579:i32)
                      }
                    }
                  }
                }
              }
              frame 5 {
                # "读取标定状态"
                n206 = call "发送读取指定ID帧.vi"("T_ID"=w592, "R_ID"=w590, "CAN_Frame"="04 31 03 33 01 00 00 00", "error in (no error)"=w591) -> ("OK"=w588:bool, "Out_Time"=w587:bool, "Recive"=w583:u8[], "error out"=w585:errorcluster)  [unwired: 7 in, 1 out]
                n207 = case shown="真" w588 {
                  tunnel: w587 -> [w596 _]
                  tunnel: [TRUE w602] -> w586
                  tunnel: w585 -> [w594 w611]
                  tunnel: [w593 w611] -> w584
                  tunnel: w583 -> [_ w608]
                  tunnel: w582 -> [_ w604]
                  tunnel: [_ w603] -> w581
                  frame False {
                    n208 = local write "Out_Time"(w596) -> ()
                    n209 = call <vilib>:"Simple Error Handler.vi"("error in (no error)"=w594) -> ("error out"=w593:errorcluster)  [unwired: 4 in, 4 out]
                  }
                  frame True {
                    n210 = Split 1D Array(array=w608, index=5 ("索引")) -> (first subarray=w606:u8[], second subarray=w599:u8[])
                    n211 = Equal?(x=w606, y=u8[] [5, 113, 3, 51, 1]) -> (x = y?=w609:bool[])
                    n212 = Index Array(array=w599) -> (element=w601:u8)  [unwired: 1 in]
                    n213 = And Array Elements(Boolean array=w609) -> (logical AND=w605:bool)
                    n214 = Equal?(x=w601, y=u8 1 ("数值")) -> (x = y?=w597:bool)
                    n215 = Compound Arithmetic op=AND ("复合运算")(w605, w597) -> (w598:bool)
                    n216 = case shown="真" w598 {
                      selector: w598 -> [_ w615]
                      tunnel: w604 -> [w612 w617]
                      tunnel: [w612 w616] -> w603
                      tunnel: [TRUE _] -> w602
                      frame False {
                      }
                      frame True {
                        n217 = local write "标定成功"(w615) -> ()
                        n218 = Increment(x=w617) -> (x+1=w616:i32)
                        n219 = call "浮动通知.vi"("通知内容"="扭矩标定成功") -> ()  [unwired: 11 in]
                      }
                    }
                  }
                }
              }
              frame 6 {
                # "复位MCU"
                n220 = call "发送读取指定ID帧.vi"("T_ID"=w629, "R_ID"=w627, "CAN_Frame"="02 11 01 00 00 00 00 00", "error in (no error)"=w628) -> ("OK"=w625:bool, "Out_Time"=w624:bool, "Recive"=w620:u8[], "error out"=w622:errorcluster)  [unwired: 7 in, 1 out]
                n221 = case shown="真" w625 {
                  tunnel: w624 -> [w633 _]
                  tunnel: [TRUE w634] -> w623
                  tunnel: w622 -> [w631 w641]
                  tunnel: [w630 w641] -> w621
                  tunnel: w620 -> [_ w638]
                  tunnel: w619 -> [_ w637]
                  tunnel: [_ w636] -> w618
                  frame False {
                    n222 = local write "Out_Time"(w633) -> ()
                    n223 = call <vilib>:"Simple Error Handler.vi"("error in (no error)"=w631) -> ("error out"=w630:errorcluster)  [unwired: 4 in, 4 out]
                  }
                  frame True {
                    n224 = Equal?(x=w638, y=u8[] [2, 81, 1, 0, 0, 0, 0, 0]) -> (x = y?=w639:bool[])
                    n225 = And Array Elements(Boolean array=w639) -> (logical AND=w635:bool)
                    n226 = case shown="真" w635 {
                      selector: w635 -> [_ w645]
                      tunnel: w637 -> [w643 w647]
                      tunnel: [w643 w646] -> w636
                      tunnel: [TRUE FALSE] -> w634
                      frame False {
                      }
                      frame True {
                        n227 = local write "完成"(w645) -> ()
                        n228 = Increment(x=w647) -> (x+1=w646:i32)
                      }
                    }
                  }
                }
              }
              frame 7 {
                # "等待MCU重启"
                n229 = call "浮动通知.vi"("通知内容"="扭矩已标定") -> ()  [unwired: 11 in]
                n230 = Wait (ms)(milliseconds to wait=u32 1000 ("等待时间（毫秒）")) -> ()  [unwired: 1 out]
                n231 = Increment(x=w651) -> (x+1=w650:i32)
              }
            }
          }
        }
        frame "扭矩标定清除" {
          w658 = 0  # Step
          n232 = while {
            tunnel: w655 -> [w665]
            tunnel: w654 -> [w663]
            shift-right: [w659] -> _
            shift-left: w658 -> [w662]
            shift-right: [w660] -> w656
            shift-left: w657 -> [w664]
            stop <- w661 stop-if-true
            n233 = case shown="1" w662 {
              selector: w662 -> [w672 w686]
              tunnel: w665 -> [w675 w685]
              tunnel: w664 -> [w667 w687]
              tunnel: w663 -> [w674 w688]
              tunnel: [w670 w683] -> w661
              tunnel: [w669 w682] -> w660
              tunnel: [w671 w684] -> w659
              frame 0, Default {
                # "进入扩展服务"
                n234 = call "扩展会话.vi"("error in"=w667, "R_ID"=w674, "T_ID"=w675) -> ("error out"=w666:errorcluster, "OK"=w673:bool)  [unwired: 7 in]
                n235 = case shown="真" w673 {
                  tunnel: w672 -> [w678 w681]
                  tunnel: [w678 w680] -> w671
                  tunnel: [TRUE _] -> w670
                  tunnel: [w676 w679] -> w669
                  tunnel: w666 -> [w676 w679]
                  frame False {
                  }
                  frame True {
                    n236 = Increment(x=w681) -> (x+1=w680:i32)
                  }
                }
                n237 = call "浮动通知.vi"("通知内容"="扭矩标定清除") -> ()  [unwired: 11 in]
              }
              frame 1 {
                # "启动转角标定清除"
                n238 = call "发送读取指定ID帧.vi"("T_ID"=w685, "R_ID"=w688, "CAN_Frame"="04 2E 07 05 01 00 00 00", "error in (no error)"=w687) -> ("OK"=w693:bool, "Out_Time"=w692:bool, "Recive"=w690:u8[], "error out"=w691:errorcluster)  [unwired: 7 in, 1 out]
                n239 = case shown="真" w693 {
                  tunnel: w692 -> [w697 _]
                  tunnel: [TRUE w698] -> w683
                  tunnel: w691 -> [w695 w705]
                  tunnel: [w694 w705] -> w682
                  tunnel: w690 -> [_ w702]
                  tunnel: w686 -> [_ w700]
                  tunnel: [_ w699] -> w684
                  frame False {
                    n240 = local write "Out_Time"(w697) -> ()
                    n241 = call <vilib>:"Simple Error Handler.vi"("error in (no error)"=w695) -> ("error out"=w694:errorcluster)  [unwired: 4 in, 4 out]
                  }
                  frame True {
                    n242 = Equal?(x=w702, y=u8[] [3, 110, 7, 5, 0, 0, 0, 0]) -> (x = y?=w703:bool[])
                    n243 = And Array Elements(Boolean array=w703) -> (logical AND=w701:bool)
                    n244 = case shown="真" w701 {
                      selector: w701 -> [_ w708]
                      tunnel: w700 -> [w707 w710]
                      tunnel: [w707 w709] -> w699
                      tunnel: [TRUE w708] -> w698
                      frame False {
                      }
                      frame True {
                        n245 = local write "完成"(w708) -> ()
                        n246 = local write "标定成功"(w708) -> ()
                        n247 = Increment(x=w710) -> (x+1=w709:i32)
                      }
                    }
                  }
                }
              }
            }
          }
        }
        frame "内部软件版本号" {
        }
        frame "客户软件版本号" {
        }
      }
      "error out" <- w27
    }
    frame #6 {
      n248 = call "点火.vi"("点火"=FALSE) -> ()  [unwired: 10 in, 1 out]
      n249 = global read "Global.vi" "Log"() -> (→"Logs":string)
    }
  }
